vi "Type-Cast-Demo.vi"() -> ()   [LabVIEW 2020]
panel:
  out "Boolean array 4":bool[](array[boolean])
  out "*(type *) &x 6":string
  out "number 2":u32
  out "*(type *) &x 5":string
  in  "Input Array":bool[](array[boolean])
  out "*(type *) &x 4":string
  in  "Boolean array 3":bool[](array[boolean])
  out "*(type *) &x 3":string
  out "*(type *) &x 2":string
  out "hex integer string":string
  out "number":u32
  out "*(type *) &x":string
  out "Boolean array 2":bool[](array[boolean])
  out "Boolean array":bool[](array[boolean])
  out "Hex 2":u32 format="%8x"
  in  "Numeric 2":sgl=135.9
  out "Numeric":sgl
  in  "Hex":u32=1124591206 format="%8x"
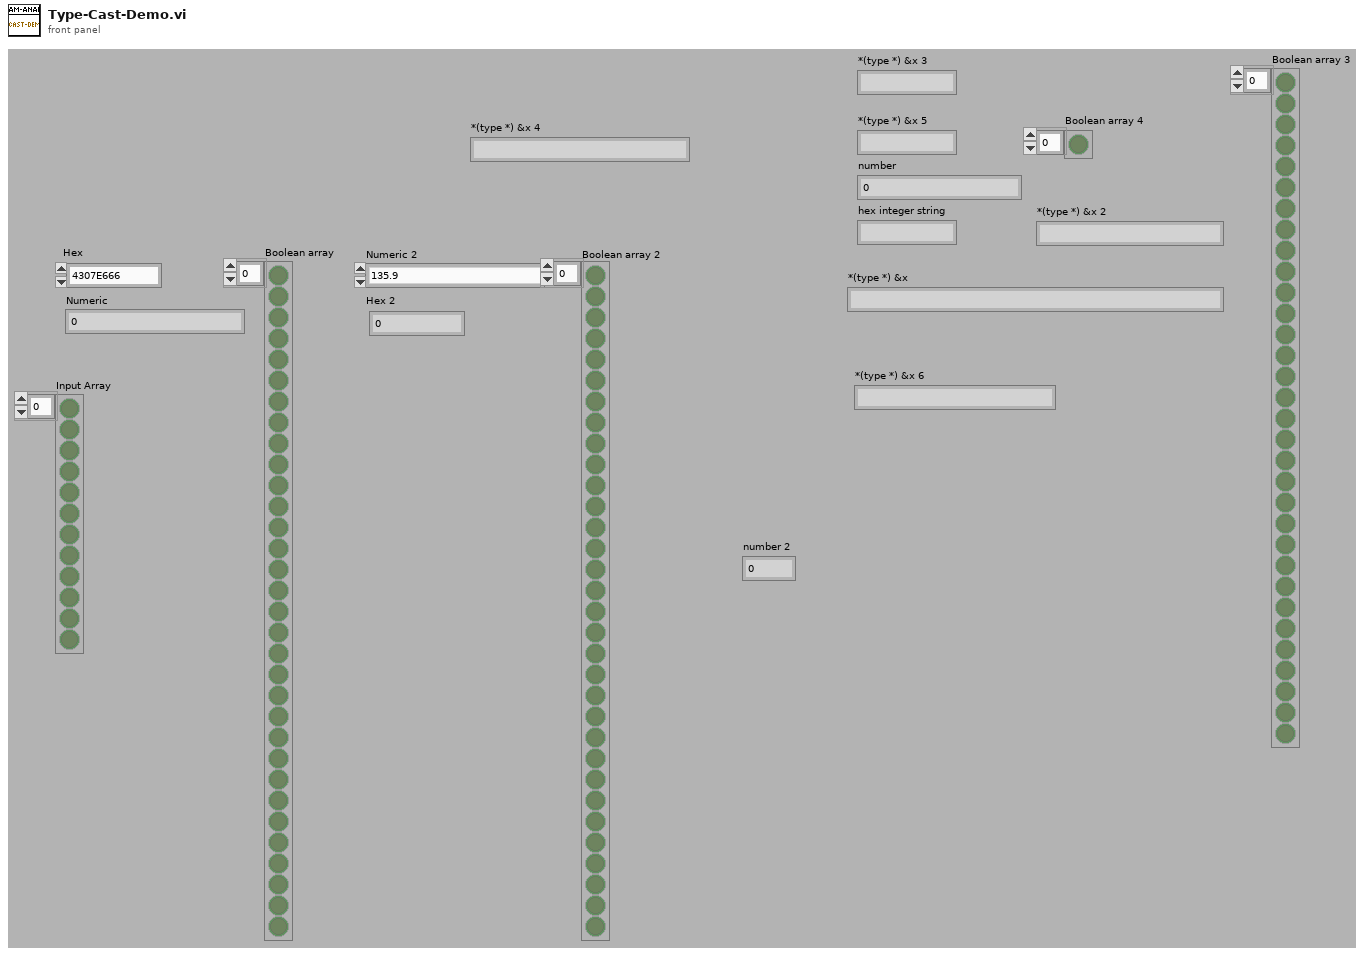
[diagram p1: front panel]
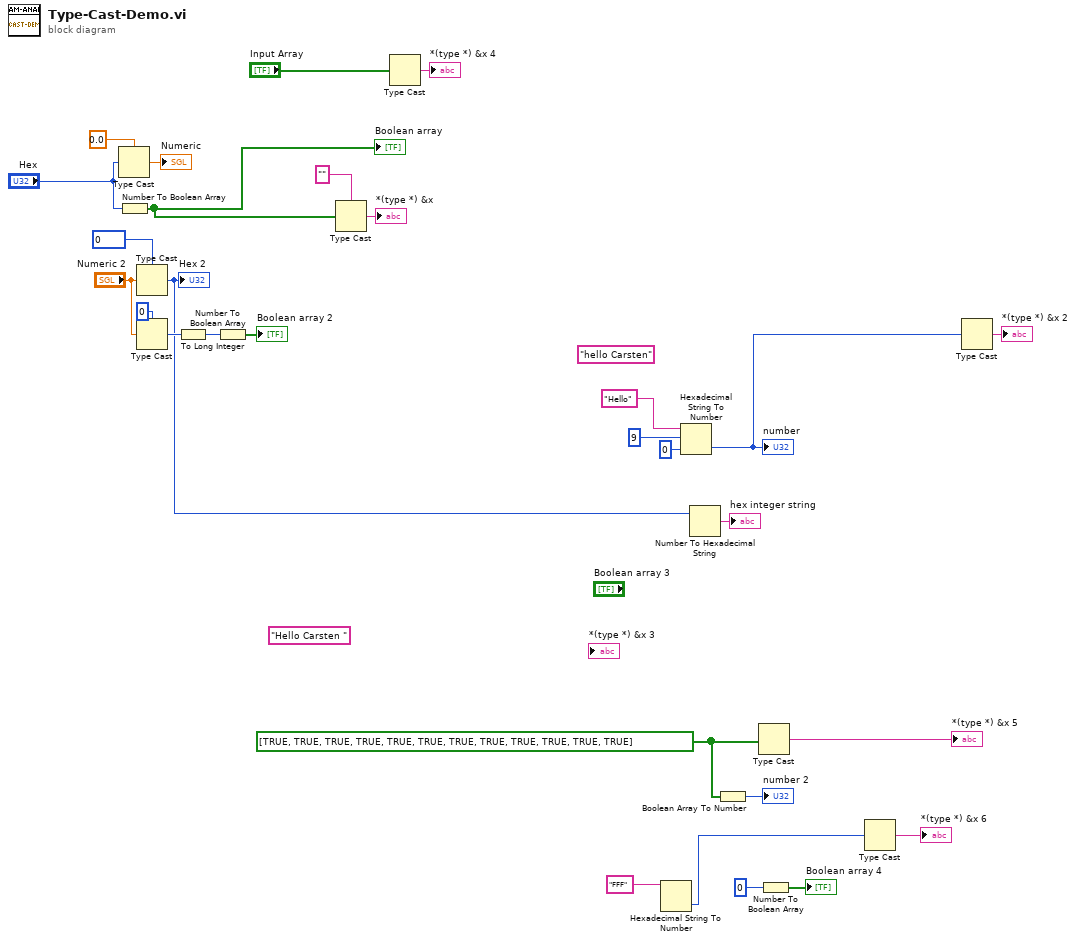
[diagram p0: block diagram]
diagram:
  w9 = bool[] [TRUE, TRUE, TRUE, TRUE, TRUE, TRUE, TRUE, TRUE, TRUE, TRUE, TRUE, TRUE] ("*(type *) &x")
  (unwired) "Hello Carsten "
  (unwired) "hello Carsten"
  n1 = Type Cast(type=sgl 0.0 ("Numeric"), x="Hex") -> (*(type *) &x=→"Numeric":sgl)
  n2 = Number To Boolean Array(number="Hex") -> (Boolean array=w13:bool[])
  "Boolean array" <- w13
  n3 = Type Cast(type=u32 0 ("Hex 2"), x="Numeric 2") -> (*(type *) &x=w20:u32)
  "Hex 2" <- w20
  n4 = Type Cast(type=0, x="Numeric 2") -> (*(type *) &x=w23:i32)
  n5 = To Long Integer(number=w23) -> (32bit integer=w24:i32)
  n6 = Number To Boolean Array(number=w24) -> (Boolean array=→"Boolean array 2":bool[])
  n7 = Type Cast(type="", x=w13) -> (*(type *) &x=→"*(type *) &x":string)
  n8 = Type Cast(x="Input Array") -> (*(type *) &x=→"*(type *) &x 4":string)  [unwired: 1 in]
  n9 = Hexadecimal String To Number(string="FFF" ("String")) -> (number=w1:u32)  [unwired: 2 in, 1 out]
  n10 = Hexadecimal String To Number(string="Hello", offset=9, default (0uL)=u32 0 ("default (0 U32)")) -> (number=w16:u32)  [unwired: 1 out]
  "number" <- w16
  n11 = Number To Hexadecimal String(2:w20) -> (0:→"hex integer string":string)  [unwired: 1 in]
  n12 = Boolean Array To Number(Boolean array=w9) -> (number=→"number 2":u32)
  n13 = Type Cast(x=w9) -> (*(type *) &x=→"*(type *) &x 5":string)  [unwired: 1 in]
  n14 = Number To Boolean Array(number=u32 0) -> (Boolean array=→"Boolean array 4":bool[])
  n15 = Type Cast(x=w1) -> (*(type *) &x=→"*(type *) &x 6":string)  [unwired: 1 in]
  n16 = Type Cast(x=w16) -> (*(type *) &x=→"*(type *) &x 2":string)  [unwired: 1 in]
